vi "set_data_for_channel.vi"(8 "error in (no error)":errorcluster, 10 "data":dbl[](array[numeric]), 11 "DAQmxWriteSignals in":refnum<class "SignalWriterMM140725DAQmx.lvclass">) -> (0 "error out":errorcluster, 3 "DAQmxWriteSignals out":refnum<class "SignalWriterMM140725DAQmx.lvclass">)   [LabVIEW 2010, in "SignalWriterMM140725DAQmx.lvclass"]
uses:
  SignalWriterMM140725DAQmx.lvclass
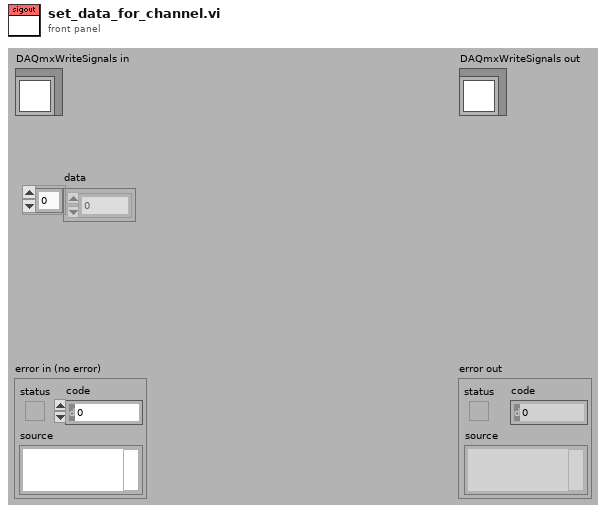
[diagram p1: front panel]
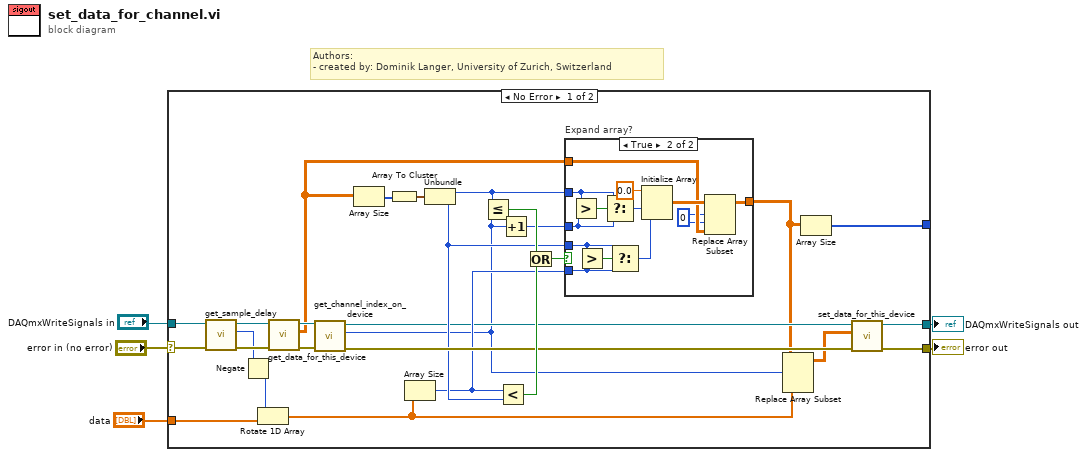
[diagram p0: block diagram]
diagram:
  # "Authors: \n- created by: Dominik Langer, University of Zurich, Switzerland"
  n1 = case shown="No Error" "error in (no error)" {
    selector: "error in (no error)" -> [w28 w49]
    tunnel: [w31 w49] -> w2
    tunnel: [w30 w48] -> w5
    tunnel: "DAQmxWriteSignals in" -> [w26 w48]
    tunnel: "data" -> [w29 _]
    tunnel: [w11 _] -> _
    frame No Error {
      n2 = call-dynamic "get_sample_delay.vi"("error in (no error)"=w28, "GenericWriteSignals in"=w26) -> ("error out"=w27:errorcluster, "sample delay (samples)"=w6:i32, "GenericWriteSignals out"=w25:refnum<class "SignalWriterMM140725DAQmx.lvclass">)  [unwired: 7 out]
      n3 = Negate(x=w6) -> (-x=w7:i32)
      n4 = Rotate 1D Array(1:w29, 2:w7) -> (0:w22:dbl[])
      n5 = call-dynamic "get_data_for_this_device.vi"("error in (no error)"=w27, "DAQmxWriteSignals in"=w25) -> ("error out"=w32:errorcluster, "data"=w8:dbl[][], "DAQmxWriteSignals out"=w33:refnum<class "SignalWriterMM140725DAQmx.lvclass">)  [unwired: 7 out]
      n6 = call-dynamic "get_channel_index_on_device.vi"("error in (no error)"=w32, "DAQmxWriteSignals.lvclass in"=w33) -> ("error out"=w19:errorcluster, "channel index on device"=w10:i32, "DAQmxWriteSignals.lvclass out"=w13:refnum<class "SignalWriterMM140725DAQmx.lvclass">)  [unwired: 7 out]
      n7 = Array Size(array=w8) -> (size(s)=w24:i32[])
      n8 = Array To Cluster(array=w24) -> (cluster=w23:cluster{"[0]":i32, "[1]":i32})
      n9 = Array Size(array=w22) -> (size(s)=w15:i32)
      n10 = Unbundle(w23) -> ("[0]"=w18:i32, "[1]"=w16:i32)
      n11 = Less Or Equal?(x=w18, y=w10) -> (x <= y?=w21:bool)
      n12 = Less?(x=w15, y=w16) -> (x < y?=w20:bool)
      n13 = Increment(x=w10) -> (x+1=w17:i32)
      n14 = Or(x=w21, y=w20) -> (x .or. y?=w14:bool)
      n15 = case "Expand array?" shown="True" w14 {
        tunnel: w18 -> [_ w45]
        tunnel: w17 -> [_ w39]
        tunnel: w16 -> [_ w42]
        tunnel: w15 -> [_ w41]
        tunnel: w8 -> [w34 w37]
        tunnel: [w34 w35] -> w12
        frame False {
        }
        frame True {
          w36 = 0 ("index (row)")
          n16 = Greater?(x=w45, y=w39) -> (0:w46:bool)
          n17 = Greater?(x=w42, y=w41) -> (0:w43:bool)
          n18 = Select(t=w45, s=w46, f=w39) -> (s? t:f=w44:i32)
          n19 = Select(t=w42, s=w43, f=w41) -> (s? t:f=w40:i32)
          n20 = Initialize Array(0.0 ("element"), w44, w40) -> (w38:dbl[][])
          n21 = Replace Array Subset(array=w38, new element=w37, index (row)=w36, index (col)=w36) -> (w35:dbl[][])
        }
      }
      n22 = Replace Array Subset(array=w12, new element=w22, index (row)=w10) -> (w9:dbl[][])  [unwired: 1 in]
      n23 = Array Size(array=w12) -> (size(s)=w11:i32[])
      n24 = call-dynamic "set_data_for_this_device.vi"("error in (no error)"=w19, "data"=w9, "DAQmxWriteSignals in"=w13) -> ("error out"=w31:errorcluster, "DAQmxWriteSignals out"=w30:refnum<class "SignalWriterMM140725DAQmx.lvclass">)  [unwired: 7 out]
    }
    frame Error {
    }
  }
  "error out" <- w2
  "DAQmxWriteSignals out" <- w5
